vi "Cleanup.vi"(8 "error in (no error)":errorcluster, 11 "TCPConfigPanel in":refnum<class "TCPConfigPanel.lvclass">) -> (0 "error out":errorcluster)   [LabVIEW 2020, in "LV-Term.lvlib" / "TCPConfigPanel.lvclass"]
uses:
  TCPConfigPanel.lvclass
  TCPConfigPanel.lvclass/TCPConfigPanel.ctl
  <vilib>/IlluminatedG/IG OOPanel/OOPanel/Panel/Panel.lvclass
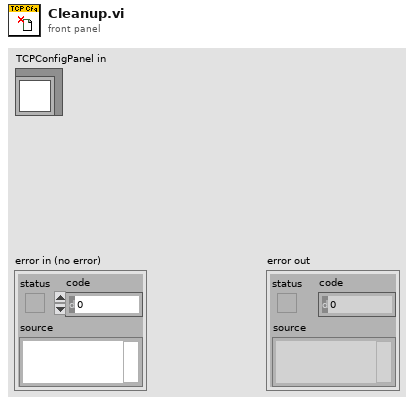
[diagram p1: front panel]
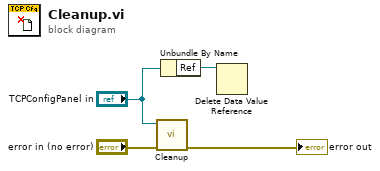
[diagram p0: block diagram]
diagram:
  n1 = call-parent "Cleanup.vi"("error in (no error)"="error in (no error)", "Panel in"="TCPConfigPanel in") -> ("error out"=→"error out":errorcluster)  [unwired: 9 in]
  n2 = Unbundle By Name("TCPConfigPanel in") -> ("Ref"=w1:refnum<data-value>)
  n3 = Delete Data Value Reference(data value reference=w1) -> ()  [unwired: 1 in, 2 out]
